vi "Hw Device list.vi"(8 "error in (no error)":errorcluster) -> (0 "error out":errorcluster, 3 "Channel List":T1)   [LabVIEW 2022 SP3]
uses:
  <resource>/objmgr/daqmx.rc
  b5ac99f9-5173-4c31-8a28-ef8ad511105c.vi
  fb49c12b-b483-4571-b40d-ecaa8db585a3.vi
  68205be7-741a-4ef4-8ff5-1684b69be710.vi
  1e1b64d9-6d49-45cf-9d80-2436e3cb3542.vi
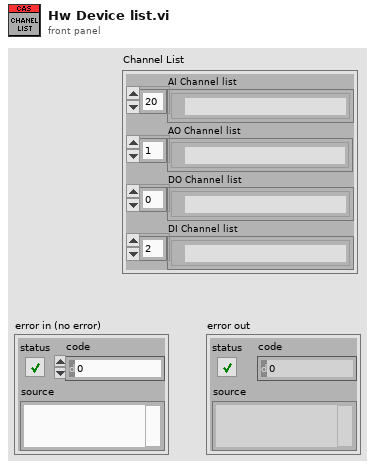
[diagram p1: front panel]
types:
  T1 = cluster{"AI Channel list":tag[], "AO Channel list":tag[], "DO Channel list ":tag[], "DI Channel list":tag[]}
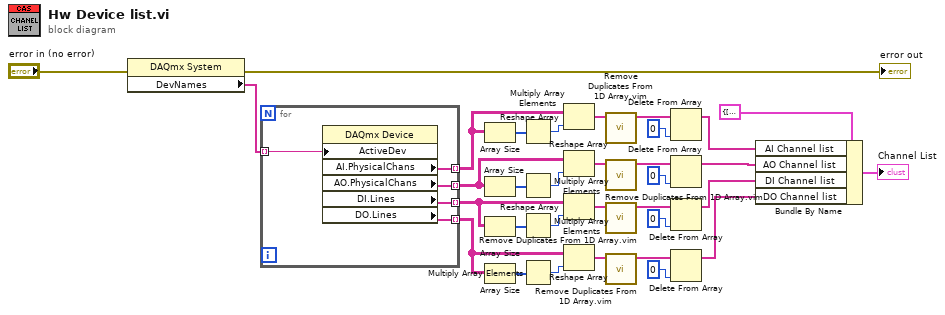
[diagram p0: block diagram]
diagram:
  n1 = property class="DAQmx System"(error in="error in (no error)") -> (error out=→"error out":errorcluster, "DevNames"=w33:tag[])  [unwired: 1 in, 1 out]
  n2 = for {
    tunnel: w33 -> [w36] mode=indexing
    tunnel: [w38] -> w28 mode=indexing
    tunnel: [w37] -> w23 mode=indexing
    tunnel: [w35] -> w14 mode=indexing
    tunnel: [w34] -> w13 mode=indexing
    n3 = property class="DAQmx Device"("ActiveDev"=w36) -> ("AI.PhysicalChans"=w38:tag[], "AO.PhysicalChans"=w37:tag[], "DI.Lines"=w35:tag[], "DO.Lines"=w34:tag[])  [unwired: 2 in, 2 out]
  }
  n4 = Array Size(array=w28) -> (size(s)=w32:i32[])
  n5 = Array Size(array=w23) -> (size(s)=w27:i32[])
  n6 = Array Size(array=w14) -> (size(s)=w22:i32[])
  n7 = Array Size(array=w13) -> (size(s)=w18:i32[])
  n8 = Multiply Array Elements(1:w32) -> (0:w31:i32)
  n9 = Multiply Array Elements(1:w27) -> (0:w26:i32)
  n10 = Multiply Array Elements(1:w22) -> (0:w21:i32)
  n11 = Multiply Array Elements(1:w18) -> (0:w17:i32)
  n12 = Reshape Array(w28, w31) -> (w30:tag[])
  n13 = Reshape Array(w23, w26) -> (w25:tag[])
  n14 = Reshape Array(w14, w21) -> (w20:tag[])
  n15 = Reshape Array(w13, w17) -> (w16:tag[])
  n16 = call "Remove Duplicates From 1D Array.vim"("array"=w30) -> ("array with duplicates removed"=w29:tag[])  [unwired: 10 in]
  n17 = call "Remove Duplicates From 1D Array.vim"("array"=w25) -> ("array with duplicates removed"=w24:tag[])  [unwired: 10 in]
  n18 = call "Remove Duplicates From 1D Array.vim"("array"=w20) -> ("array with duplicates removed"=w19:tag[])  [unwired: 10 in]
  n19 = call "Remove Duplicates From 1D Array.vim"("array"=w16) -> ("array with duplicates removed"=w15:tag[])  [unwired: 10 in]
  n20 = Delete From Array(array=w29, index=0) -> (array with subset deleted=w5:tag[])  [unwired: 1 in, 1 out]
  n21 = Delete From Array(array=w24, index=0) -> (array with subset deleted=w4:tag[])  [unwired: 1 in, 1 out]
  n22 = Delete From Array(array=w19, index=0) -> (array with subset deleted=w3:tag[])  [unwired: 1 in, 1 out]
  n23 = Delete From Array(array=w15, index=0) -> (array with subset deleted=w2:tag[])  [unwired: 1 in, 1 out]
  n24 = Bundle By Name(cluster=T1 {"AI Channel list"=[], "AO Channel list"=[], "DO Channel list "=[], "DI Channel list"=[]} ("Cluster"), "AI Channel list"=w5, "AO Channel list"=w4, "DI Channel list"=w3, "DO Channel list"=w2) -> (→"Channel List":T1)
